vi "Autonomous Independent.vi"   [LabVIEW 2015]
doc: "This VI is called when autonomous begins, and will automatically be terminated when autonomous ends. You can carry out timed or sensor driven robot movement independently without needing to return to the caller."
uses:
  AppleScript/AppleScript Global Data.vi
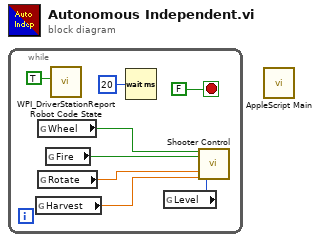
[diagram p0: block diagram]
diagram:
  n1 = while {
    stop <- FALSE stop-if-true
    n2 = global read "AppleScript Global Data.vi" "Harvest"() -> (w2:dbl)
    n3 = global read "AppleScript Global Data.vi" "Wheel"() -> (w5:bool)
    n4 = global read "AppleScript Global Data.vi" "Rotate"() -> (w3:dbl)
    n5 = global read "AppleScript Global Data.vi" "Fire"() -> (w4:bool)
    n6 = call <vilib>:"WPI_DriverStationReport Robot Code State.vi"("Autonomous"=TRUE) -> ()  [unwired: 10 in, 1 out]
    n7 = Wait (ms)(milliseconds to wait=u32 20) -> ()  [unwired: 1 out]
    n8 = global read "AppleScript Global Data.vi" "Level"() -> (w1:i32)
    n9 = call "Shooter Control.vi"("Shooter Wheel On?"=w5, "Fire"=w4, "Rotate Tweak"=w3, "Harvester Axis"=w2, "Shooter Arm Level"=w1) -> ()  [unwired: 15 in]
  }
  n10 = call "AppleScript Main.vi"() -> ()  [unwired: 12 in]
